vi "Define DataTable Columns.vi"(8 "error in (no error)":errorcluster, 9 "ReadOnly":bool, 10 "ColumnSetup":T1[](array[typedef]) {"MinWidth" min=2 step=1; "AutoSizeMode" items=["None"=1, "ColumnHeader"=2, "AllCellsExceptHeader"=4, "AllCells"=6, "DisplayedCellsExceptHeader"=8, "DisplayedCells"=10, "Fill"=16]; "FillWeight" min=1 max=100}, 11 "DataTable In":refnum<class "DataTable.lvclass">) -> (0 "error out":errorcluster, 3 "DataTable Out":refnum<class "DataTable.lvclass">)   [LabVIEW 2016, in "DataGrid.lvlib" / "DataTable.lvclass"]
doc: "Defines the columns of the dataTable that is used to store all display data. If called more than once, it will add columns to the existing dataTable, so resulting in more (possibly duplicate) columns."
uses:
  <userlib>/LabVIEWdotNetDataGrid/source/DataTable/DataTable.lvclass
  <userlib>/LabVIEWdotNetDataGrid/source/GridColumn/ColumnDefinition.ctl
  <userlib>/LabVIEWdotNetDataGrid/source/GridColumn/ColumnType.ctl
  <userlib>/LabVIEWdotNetDataGrid/source/DataTable/DataTable.lvclass/DataTable.ctl
  System.Data
  <userlib>/LabVIEWdotNetDataGrid/source/DataTable/Read DataTable.vi
  <userlib>/LabVIEWdotNetDataGrid/source/GridColumn/GridColumn.lvclass
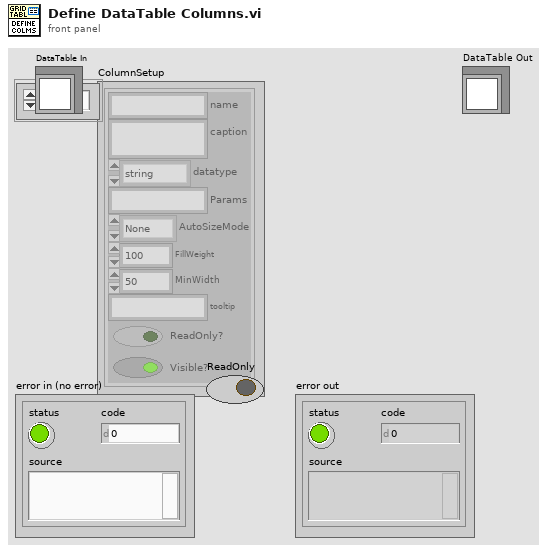
[diagram p1: front panel]
types:
  T1 = typedef "DataGrid.lvlib/GridColumn.lvclass/ColumnDefinition.ctl" = cluster{"name":string, "caption":string, "datatype":T2, "Params":string, "AutoSizeMode":i32, "FillWeight":sgl, "MinWidth":u32, "tooltip":string, "ReadOnly?":bool, "Visible?":bool}
  T2 = typedef "DataGrid.lvlib/GridColumn.lvclass/ColumnType.ctl" = enum16{"string", "image", "check", "numeric", "timestamp", "button", "combo", "link"}
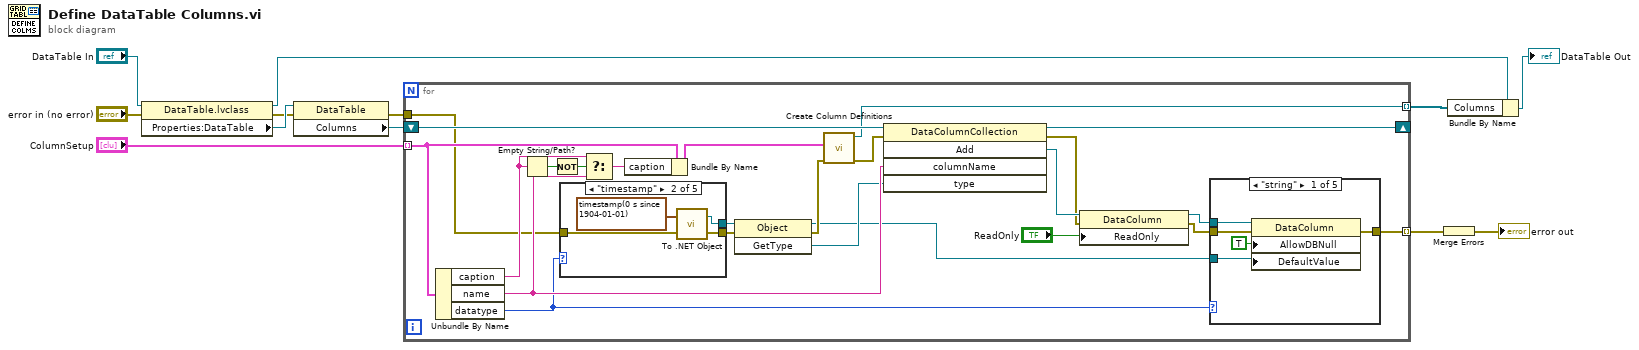
[diagram p0: block diagram]
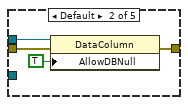
[diagram p2: hidden frame]
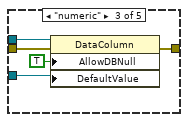
[diagram p3: hidden frame]
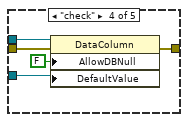
[diagram p4: hidden frame]
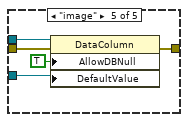
[diagram p5: hidden frame]
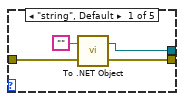
[diagram p6: hidden frame]
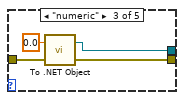
[diagram p7: hidden frame]
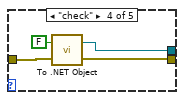
[diagram p8: hidden frame]
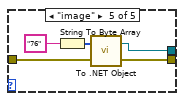
[diagram p9: hidden frame]
diagram:
  n1 = property class="DataTable.lvclass"(reference="DataTable In", error in="error in (no error)") -> (reference out=w6:refnum<class "DataTable.lvclass">, error out=w2:errorcluster, "Properties:DataTable"=w9:refnum<k24>)
  n2 = property class="DataTable"(reference=w9, error in=w2) -> (error out=w1:errorcluster, "Columns"=w8:refnum<k24>)  [unwired: 1 out]
  n3 = for {
    tunnel: "ColumnSetup" -> [w30] mode=indexing
    tunnel: [w35] -> w10 mode=indexing
    shift-right: [w27] -> _
    shift-left: w8 -> [w34]
    tunnel: [w33] -> w4 mode=indexing
    tunnel: w1 -> [w14]
    n4 = Unbundle By Name(w30) -> ("caption"=w28:string, "name"=w24:string, "datatype"=w13:T2)
    n5 = Empty String/Path?(string/path=w28) -> (empty?=w32:bool)
    n6 = Not(x=w32) -> (.not. x?=w15:bool)
    n7 = case shown="\"timestamp\"" w13 {
      tunnel: [w63 w67 w71 w75 w79] -> w23
      tunnel: [w62 w66 w70 w74 w78] -> w21
      tunnel: w14 -> [w61 w65 w69 w73 w77]
      frame "string", Default {
        n8 = call <vilib>:"To .NET Object.vi"("error in (no error)"=w61, "anything"="" ("name")) -> ("error out"=w62:errorcluster, ".NET object"=w63:refnum<k24>)
      }
      frame "timestamp" {
        n9 = call <vilib>:"To .NET Object.vi"("error in (no error)"=w65, "anything"=timestamp(0 s since 1904-01-01) ("name")) -> ("error out"=w66:errorcluster, ".NET object"=w67:refnum<k24>)
      }
      frame "numeric" {
        n10 = call <vilib>:"To .NET Object.vi"("error in (no error)"=w69, "anything"=0.0 ("name")) -> ("error out"=w70:errorcluster, ".NET object"=w71:refnum<k24>)
      }
      frame "check" {
        n11 = call <vilib>:"To .NET Object.vi"("error in (no error)"=w73, "anything"=FALSE) -> ("error out"=w74:errorcluster, ".NET object"=w75:refnum<k24>)
      }
      frame "image" {
        n12 = String To Byte Array(string="76") -> (unsigned byte array=w81:u8[])
        n13 = call <vilib>:"To .NET Object.vi"("error in (no error)"=w77, "anything"=w81) -> ("error out"=w78:errorcluster, ".NET object"=w79:refnum<k24>)
      }
    }
    n14 = Select(t=w28, s=w15, f=w24) -> (s? t:f=w31:string)
    n15 = Bundle By Name(cluster=w30, "caption"=w31) -> (w29:T1)
    n16 = invoke class="Object" method="GetType"(reference=w23, error in=w21) -> (reference out=w16:refnum<k24>, error out=w20:errorcluster, "GetType"=w22:refnum<k24>)  [unwired: 1 in]
    n17 = call <userlib>:"Create Column Definitions.vi"("error in (no error)"=w20, "Column"=w29) -> ("error out"=w36:errorcluster, "GridColumn out"=w33:refnum<class "GridColumn.lvclass">)  [unwired: 8 in]
    n18 = invoke class="DataColumnCollection" method="Add"(reference=w34, error in=w36, "columnName"=w24, "type"=w22) -> (reference out=w27:refnum<k24>, error out=w18:errorcluster, "Add"=w25:refnum<k24>)  [unwired: 1 in, 2 out]
    n19 = property class="DataColumn"(reference=w25, error in=w18, "ReadOnly"="ReadOnly") -> (reference out=w19:refnum<k24>, error out=w17:errorcluster)
    n20 = case shown="\"string\"" w13 {
      tunnel: w19 -> [w39 w43 w48 w53 w58]
      tunnel: w17 -> [w41 w45 w50 w55 w60]
      tunnel: [w40 w44 w49 w54 w59] -> w35
      tunnel: w16 -> [w37 _ w46 w51 w56]
      frame "string" {
        n21 = property class="DataColumn"(reference=w39, error in=w41, "AllowDBNull"=TRUE, "DefaultValue"=w37) -> (error out=w40:errorcluster)  [unwired: 1 out]
      }
      frame Default {
        n22 = property class="DataColumn"(reference=w43, error in=w45, "AllowDBNull"=TRUE) -> (error out=w44:errorcluster)  [unwired: 1 out]
      }
      frame "numeric" {
        n23 = property class="DataColumn"(reference=w48, error in=w50, "AllowDBNull"=TRUE, "DefaultValue"=w46) -> (error out=w49:errorcluster)  [unwired: 1 out]
      }
      frame "check" {
        n24 = property class="DataColumn"(reference=w53, error in=w55, "AllowDBNull"=FALSE, "DefaultValue"=w51) -> (error out=w54:errorcluster)  [unwired: 1 out]
      }
      frame "image" {
        n25 = property class="DataColumn"(reference=w58, error in=w60, "AllowDBNull"=TRUE, "DefaultValue"=w56) -> (error out=w59:errorcluster)  [unwired: 1 out]
      }
    }
  }
  n26 = Merge Errors(w10) -> (→"error out":errorcluster)
  n27 = Bundle By Name(cluster=w6, "Columns"=w4) -> (→"DataTable Out":refnum<class "DataTable.lvclass">)
